vi "ExcelBinData1.vi"(5 "step":string, 6 "start row":i32, 7 "jobno":string, 8 "error in (no error) 2":errorcluster, 9 "report in":refnum<class "NI_report.lvclass">, 10 "error in (no error)":errorcluster, 11 "connection reference 2":T1) -> (0 "error out 2":errorcluster, 1 "report out":refnum<class "NI_report.lvclass">, 2 "error out":errorcluster, 3 "connection reference":T1)   [LabVIEW 2012]
uses:
  <vilib>/addons/database/Connection.llb/Conn ObjectReference.ctl
  <vilib>/Utility/NIReport.llb/NI_report.lvclass
  <vilib>/addons/database/Auxilliary.llb/DB Tools Cursor Type.ctl
  <vilib>/addons/database/Connection.llb/Conn Execute.vi
  <vilib>/addons/database/Recordset.llb/Rec Fetch String Data (R).vi
  <vilib>/addons/database/Recordset.llb/Rec Fetch Integer Data (R).vi
  <vilib>/addons/database/Recordset.llb/Rec Destroy - Connection.vi
  <vilib>/addons/database/NI_Database_API.lvlib
  <vilib>/Utility/NIReport.llb/Excel/NI_Excel.lvclass
panel:
  in  "start (0, 0)":cluster{"start row":i32, "start column":i32}
  out "concatenated string":string
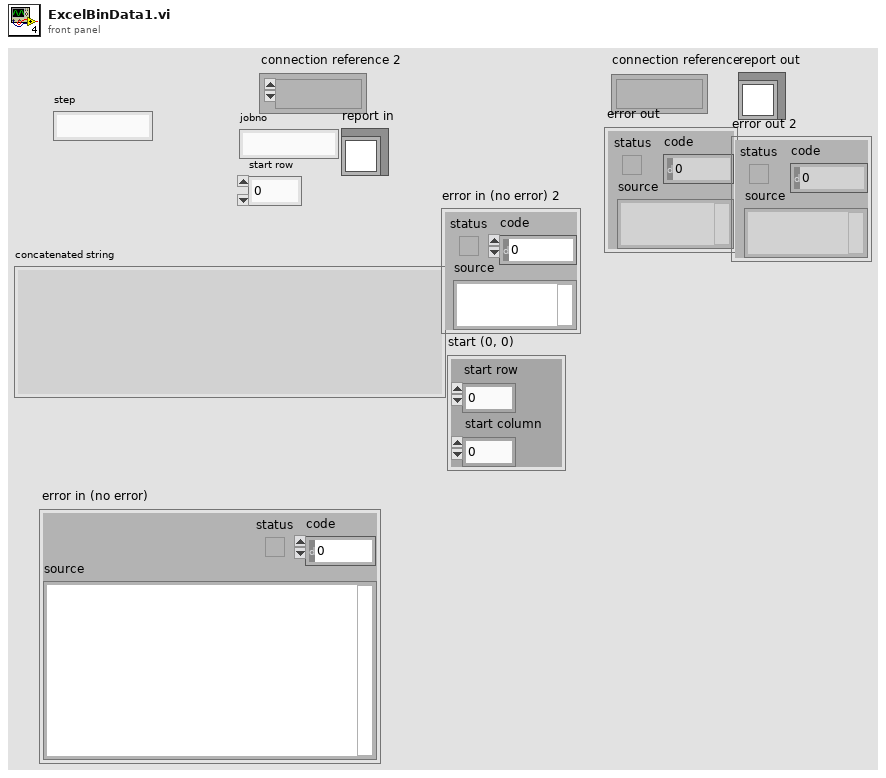
[diagram p1: front panel]
types:
  T1 = typedef "NI_Database_API.lvlib/Conn ObjectReference.ctl" = refnum<k1>
  T2 = typedef "NI_Database_API.lvlib/DB Tools Cursor Type.ctl" = enum16{"forward-only", "keyset", "dynamic", "static"}
  T3 = typedef "NI_Database_API.lvlib/Rec ObjectReference.ctl" = refnum<k1>
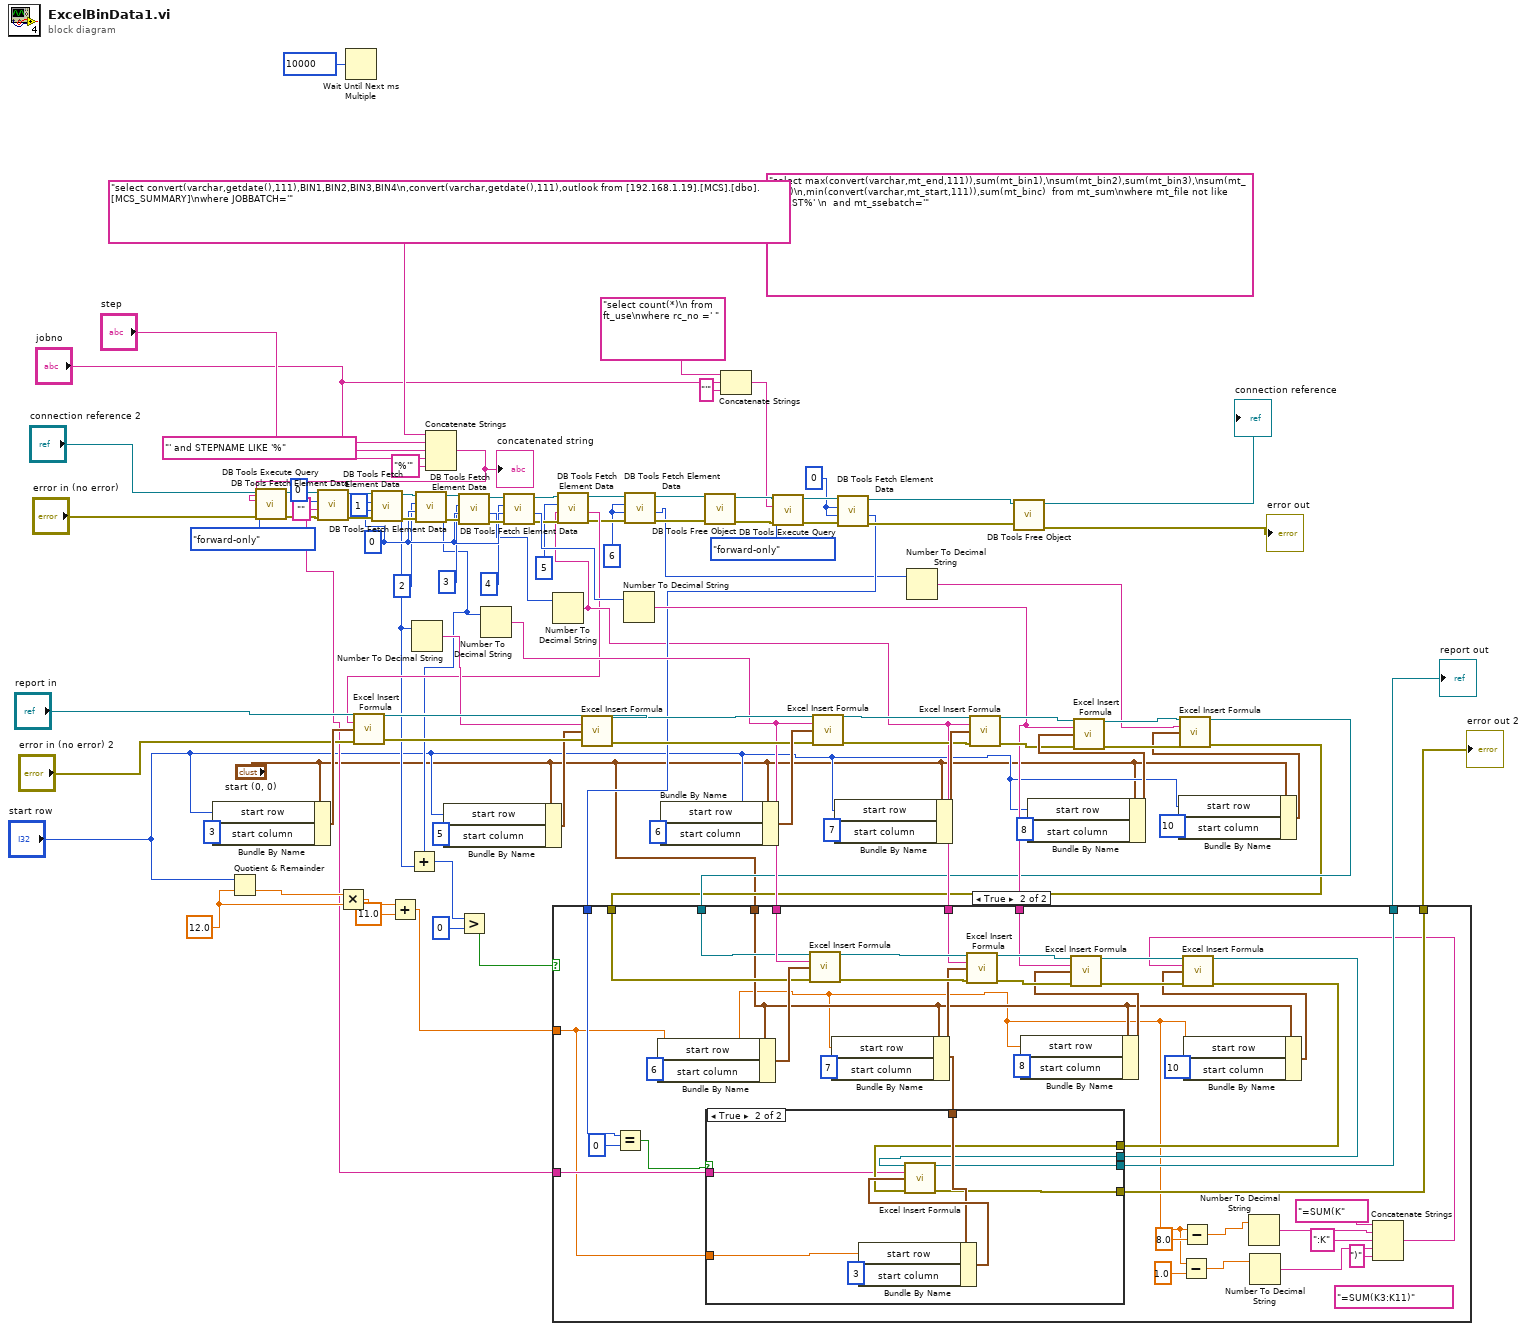
[diagram p0: block diagram]
diagram:
  (unwired) "select max(convert(varchar,mt_end,111)),sum(mt_bin1),\nsum(mt_bin2),sum(mt_bin3),\nsum(mt_bin4)\n,min(convert(varchar,mt_start,111)),sum(mt_binc)  from mt_sum\nwhere mt_file not like '%TEST%' \n  and mt_ssebatch='"
  w12 = 6
  w27 = 0
  w50 = 12.0 ("y")
  w83 = 0
  n1 = Bundle By Name(cluster="start (0, 0)", "start row"="start row", "start column"=3) -> (w78:cluster{"start row":i32, "start column":i32})
  n2 = Quotient & Remainder(x="start row", y=w50) -> (floor(x/y)=w51:dbl)  [unwired: 1 out]
  n3 = Multiply(x=w51, y=w50) -> (x*y=w49:dbl)
  n4 = Wait Until Next ms Multiple(millisecond multiple=u32 10000) -> ()  [unwired: 1 out]
  n5 = Add(x=w49, y=11.0) -> (x+y=w43:dbl)
  n6 = Concatenate Strings("select convert(varchar,getdate(),111),BIN1,BIN2,BIN3,BIN4\n,convert(varchar,getdate(),111),outlook from [192.168.1.19].[MCS].[dbo].[MCS_SUMMARY]\nwhere JOBBATCH='", "jobno", "' and STEPNAME LIKE '%" ("string"), "step", "%'" ("string")) -> (w97:string)
  "concatenated string" <- w97
  n7 = call-poly <vilib>:"DB Tools Execute Query.vi"("error in (no error)"="error in (no error)", "cursor type"=DB_Tools_Cursor_Type."forward-only", "SQL query"=w97, "connection reference"="connection reference 2") -> ("error out"=w94:errorcluster, "recordset reference"=w95:T3)  [unwired: 4 in]
  n8 = call-poly <vilib>:"DB Tools Fetch Element Data.vi"("error in (no error)"=w94, "type"="", "column index"=0, "recordset reference"=w95) -> ("error out"=w90:errorcluster, "data"=w25:string, "recordset reference out"=w91:T3)  [unwired: 3 in]
  n9 = call-poly <vilib>:"DB Tools Fetch Element Data.vi"("error in (no error)"=w90, "type"=w83, "column index"=1, "recordset reference"=w91) -> ("error out"=w86:errorcluster, "data"=w18:i32, "recordset reference out"=w89:T3)  [unwired: 3 in]
  n10 = Number To Decimal String(number=w18) -> (decimal integer string=w73:string)  [unwired: 1 in]
  n11 = call-poly <vilib>:"DB Tools Fetch Element Data.vi"("error in (no error)"=w86, "type"=w83, "column index"=2, "recordset reference"=w89) -> ("error out"=w85:errorcluster, "data"=w17:i32, "recordset reference out"=w88:T3)  [unwired: 3 in]
  n12 = Add(x=w17, y=w18) -> (x+y=w19:i32)
  n13 = Bundle By Name(cluster="start (0, 0)", "start row"="start row", "start column"=5) -> (w72:cluster{"start row":i32, "start column":i32})
  n14 = call-poly <vilib>:"DB Tools Fetch Element Data.vi"("error in (no error)"=w85, "type"=w83, "column index"=3, "recordset reference"=w88) -> ("error out"=w84:errorcluster, "data"=w67:i32, "recordset reference out"=w87:T3)  [unwired: 3 in]
  n15 = Greater?(x=w19, y=0) -> (0:w46:bool)
  n16 = Number To Decimal String(number=w17) -> (decimal integer string=w44:string)  [unwired: 1 in]
  n17 = call-poly <vilib>:"DB Tools Fetch Element Data.vi"("error in (no error)"=w84, "type"=w83, "column index"=4, "recordset reference"=w87) -> ("error out"=w23:errorcluster, "data"=w66:i32, "recordset reference out"=w24:T3)  [unwired: 3 in]
  n18 = Number To Decimal String(number=w67) -> (decimal integer string=w21:string)  [unwired: 1 in]
  n19 = call-poly <vilib>:"DB Tools Fetch Element Data.vi"("error in (no error)"=w23, "type"=w21, "column index"=5, "recordset reference"=w24) -> ("error out"=w14:errorcluster, "data"=w20:string, "recordset reference out"=w16:T3)  [unwired: 3 in]
  n20 = call <vilib>:"Excel Insert Formula.vi"("report in"="report in", "formula"=w20, "start (0, 0)"=w78, "error in (no error)"="error in (no error) 2") -> ("report out"=w76:refnum<class "NI_report.lvclass">, "error out"=w75:errorcluster)  [unwired: 10 in]
  n21 = call <vilib>:"Excel Insert Formula.vi"("report in"=w76, "formula"=w73, "start (0, 0)"=w72, "error in (no error)"=w75) -> ("report out"=w68:refnum<class "NI_report.lvclass">, "error out"=w70:errorcluster)  [unwired: 10 in]
  n22 = Number To Decimal String(number=w66) -> (decimal integer string=w45:string)  [unwired: 1 in]
  n23 = call-poly <vilib>:"DB Tools Fetch Element Data.vi"("error in (no error)"=w14, "type"=w12, "column index"=w12, "recordset reference"=w16) -> ("error out"=w13:errorcluster, "data"=w11:i32, "recordset reference out"=w15:T3)  [unwired: 3 in]
  n24 = Bundle By Name(cluster="start (0, 0)", "start row"="start row", "start column"=6) -> (w71:cluster{"start row":i32, "start column":i32})
  n25 = call-poly <vilib>:"DB Tools Free Object.vi"("error in (no error)"=w13, "recordset reference"=w15) -> ("error out"=w39:errorcluster, "connection reference"=w40:T1)  [unwired: 8 in]
  n26 = Concatenate Strings("select count(*)\n from ft_use\nwhere rc_no =' " ("string"), "jobno", "'" ("string")) -> (w28:string)
  n27 = call-poly <vilib>:"DB Tools Execute Query.vi"("error in (no error)"=w39, "cursor type"=DB_Tools_Cursor_Type."forward-only", "SQL query"=w28, "connection reference"=w40) -> ("error out"=w37:errorcluster, "recordset reference"=w38:T3)  [unwired: 4 in]
  n28 = call <vilib>:"Excel Insert Formula.vi"("report in"=w68, "formula"=w44, "start (0, 0)"=w71, "error in (no error)"=w70) -> ("report out"=w61:refnum<class "NI_report.lvclass">, "error out"=w59:errorcluster)  [unwired: 10 in]
  n29 = Bundle By Name(cluster="start (0, 0)", "start row"="start row", "start column"=7) -> (w63:cluster{"start row":i32, "start column":i32})
  n30 = call-poly <vilib>:"DB Tools Fetch Element Data.vi"("error in (no error)"=w37, "type"=w27, "column index"=w27, "recordset reference"=w38) -> ("error out"=w35:errorcluster, "data"=w26:i32, "recordset reference out"=w36:T3)  [unwired: 3 in]
  n31 = Number To Decimal String(number=w11) -> (decimal integer string=w6:string)  [unwired: 1 in]
  n32 = call <vilib>:"Excel Insert Formula.vi"("report in"=w61, "formula"=w21, "start (0, 0)"=w63, "error in (no error)"=w59) -> ("report out"=w60:refnum<class "NI_report.lvclass">, "error out"=w58:errorcluster)  [unwired: 10 in]
  n33 = call-poly <vilib>:"DB Tools Free Object.vi"("error in (no error)"=w35, "recordset reference"=w36) -> ("error out"=→"error out":errorcluster, "connection reference"=→"connection reference":T1)  [unwired: 8 in]
  n34 = Bundle By Name(cluster="start (0, 0)", "start row"="start row", "start column"=8) -> (w62:cluster{"start row":i32, "start column":i32})
  n35 = call <vilib>:"Excel Insert Formula.vi"("report in"=w60, "formula"=w45, "start (0, 0)"=w62, "error in (no error)"=w58) -> ("report out"=w10:refnum<class "NI_report.lvclass">, "error out"=w9:errorcluster)  [unwired: 10 in]
  n36 = Bundle By Name(cluster="start (0, 0)", "start row"="start row", "start column"=10) -> (w2:cluster{"start row":i32, "start column":i32})
  n37 = call <vilib>:"Excel Insert Formula.vi"("report in"=w10, "formula"=w6, "start (0, 0)"=w2, "error in (no error)"=w9) -> ("report out"=w8:refnum<class "NI_report.lvclass">, "error out"=w7:errorcluster)  [unwired: 10 in]
  n38 = case shown="True" w46 {
    tunnel: "start (0, 0)" -> [_ w115]
    tunnel: w45 -> [_ w132]
    tunnel: w21 -> [_ w131]
    tunnel: w44 -> [_ w130]
    tunnel: w43 -> [_ w110]
    tunnel: [w100 w121] -> w42
    tunnel: [w101 w122] -> w41
    tunnel: w7 -> [w101 w128]
    tunnel: w8 -> [w100 w127]
    tunnel: w26 -> [_ w126]
    tunnel: w25 -> [_ w120]
    frame False {
    }
    frame True {
      (unwired) "=SUM(K3:K11)"
      n39 = Equal?(x=w126, y=0) -> (x = y?=w124:bool)
      n40 = Bundle By Name(cluster=w115, "start row"=w110, "start column"=6) -> (w140:cluster{"start row":i32, "start column":i32})
      n41 = call <vilib>:"Excel Insert Formula.vi"("report in"=w127, "formula"=w130, "start (0, 0)"=w140, "error in (no error)"=w128) -> ("report out"=w136:refnum<class "NI_report.lvclass">, "error out"=w134:errorcluster)  [unwired: 10 in]
      n42 = Bundle By Name(cluster=w115, "start row"=w110, "start column"=7) -> (w123:cluster{"start row":i32, "start column":i32})
      n43 = call <vilib>:"Excel Insert Formula.vi"("report in"=w136, "formula"=w131, "start (0, 0)"=w123, "error in (no error)"=w134) -> ("report out"=w135:refnum<class "NI_report.lvclass">, "error out"=w133:errorcluster)  [unwired: 10 in]
      n44 = Bundle By Name(cluster=w115, "start row"=w110, "start column"=8) -> (w129:cluster{"start row":i32, "start column":i32})
      n45 = call <vilib>:"Excel Insert Formula.vi"("report in"=w135, "formula"=w132, "start (0, 0)"=w129, "error in (no error)"=w133) -> ("report out"=w119:refnum<class "NI_report.lvclass">, "error out"=w118:errorcluster)  [unwired: 10 in]
      n46 = Subtract(x=w110, y=1.0) -> (x-y=w105:dbl)
      n47 = Subtract(x=w110, y=8.0) -> (x-y=w108:dbl)
      n48 = Bundle By Name(cluster=w115, "start row"=w110, "start column"=10) -> (w113:cluster{"start row":i32, "start column":i32})
      n49 = Number To Decimal String(number=w108) -> (decimal integer string=w107:string)  [unwired: 1 in]
      n50 = Number To Decimal String(number=w105) -> (decimal integer string=w104:string)  [unwired: 1 in]
      n51 = Concatenate Strings("=SUM(K" ("string"), w107, ":K" ("string"), w104, ")" ("string")) -> (w102:string)
      n52 = call <vilib>:"Excel Insert Formula.vi"("report in"=w119, "formula"=w102, "start (0, 0)"=w113, "error in (no error)"=w118) -> ("report out"=w117:refnum<class "NI_report.lvclass">, "error out"=w116:errorcluster)  [unwired: 10 in]
      n53 = case shown="True" w124 {
        tunnel: w110 -> [_ w149]
        tunnel: w123 -> [_ w148]
        tunnel: w116 -> [w141 w147]
        tunnel: [w141 w146] -> w122
        tunnel: w117 -> [w142 w145]
        tunnel: [w142 w144] -> w121
        tunnel: w120 -> [_ w143]
        frame False {
        }
        frame True {
          n54 = Bundle By Name(cluster=w148, "start row"=w149, "start column"=3) -> (w150:cluster{"start row":i32, "start column":i32})
          n55 = call <vilib>:"Excel Insert Formula.vi"("report in"=w145, "formula"=w143, "start (0, 0)"=w150, "error in (no error)"=w147) -> ("report out"=w144:refnum<class "NI_report.lvclass">, "error out"=w146:errorcluster)  [unwired: 10 in]
        }
      }
    }
  }
  "report out" <- w42
  "error out 2" <- w41
